vi "indice mesa.vi"(4 "M6":bool, 6 "M5":bool, 7 "M1":bool, 9 "M4":bool, 10 "M3":bool, 11 "M2":bool) -> (3 "Numeric":dbl)   [LabVIEW 2015]
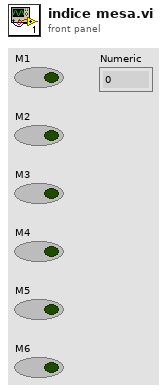
[diagram p1: front panel]
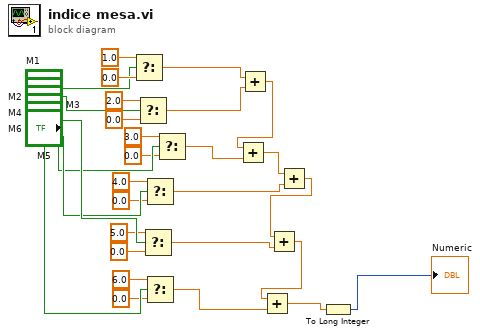
[diagram p0: block diagram]
diagram:
  n1 = Select(t=1.0, s="M1", f=0.0) -> (s? t:f=w21:dbl)
  n2 = Select(t=2.0, s="M2", f=0.0) -> (s? t:f=w22:dbl)
  n3 = Select(t=5.0, s="M5", f=0.0) -> (s? t:f=w28:dbl)
  n4 = Select(t=4.0, s="M4", f=0.0) -> (s? t:f=w26:dbl)
  n5 = Select(t=6.0, s="M6", f=0.0) -> (s? t:f=w30:dbl)
  n6 = Select(t=3.0, s="M3", f=0.0) -> (s? t:f=w24:dbl)
  n7 = Add(x=w21, y=w22) -> (x+y=w23:dbl)
  n8 = Add(x=w23, y=w24) -> (x+y=w25:dbl)
  n9 = Add(x=w25, y=w26) -> (x+y=w27:dbl)
  n10 = Add(x=w27, y=w28) -> (x+y=w29:dbl)
  n11 = Add(x=w29, y=w30) -> (x+y=w2:dbl)
  n12 = To Long Integer(number=w2) -> (32bit integer=→"Numeric":i32)
